vi "Label Targets Cones.vi"(5 "Details":bool, 7 "Annotate":bool=TRUE, 8 "Score Threshold":dbl, 9 "results":T1, 10 "Angle":dbl=53.2 format="%#_13g", 11 "Image in":T2) -> (3 "Image out":T2)   [LabVIEW 2025]
doc: "Draw scores near or on the particle and an ellipse around the target. Scores that are below the score threshold are drawn in red, above in green."
uses:
  <vilib>/vision/Image Controls.llb/IMAQ Image.ctl
  Target Fields.ctl
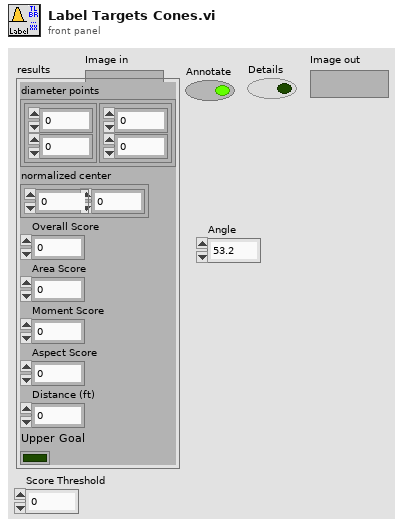
[diagram p1: front panel]
types:
  T1 = typedef "Target Fields.ctl" = cluster{"diameter points":cluster{"first point":cluster{"x":dbl, "y":dbl}, "projected point":cluster{"x":dbl, "y":dbl}}, "normalized center":cluster{"x":dbl, "y":dbl}, "Overall Score":dbl, "Area Score":dbl, "Moment Score":dbl, "Aspect Score":dbl, "Distance (ft)":dbl, "Upper Goal":bool}
  T2 = typedef "IMAQ Image.ctl" = refnum<image>
  T3 = cluster{"Desired Font (Application)":enum16{"User-specified Font", "Application Font", "System Font", "Dialog Font"}, "[User-specified Font]":cluster{"Font Name":string, "Size":i16, "Strikeout?":bool, "Italic?":bool, "Underline?":bool, "Outline?":bool, "Shadow?":bool, "Bold?":bool, "Rotation Angle":dbl}, "Horizontal Alignment":i16, "Vertical Alignment":i16}
  T4 = cluster{"first point":cluster{"x":dbl, "y":dbl}, "projected point":cluster{"x":dbl, "y":dbl}}
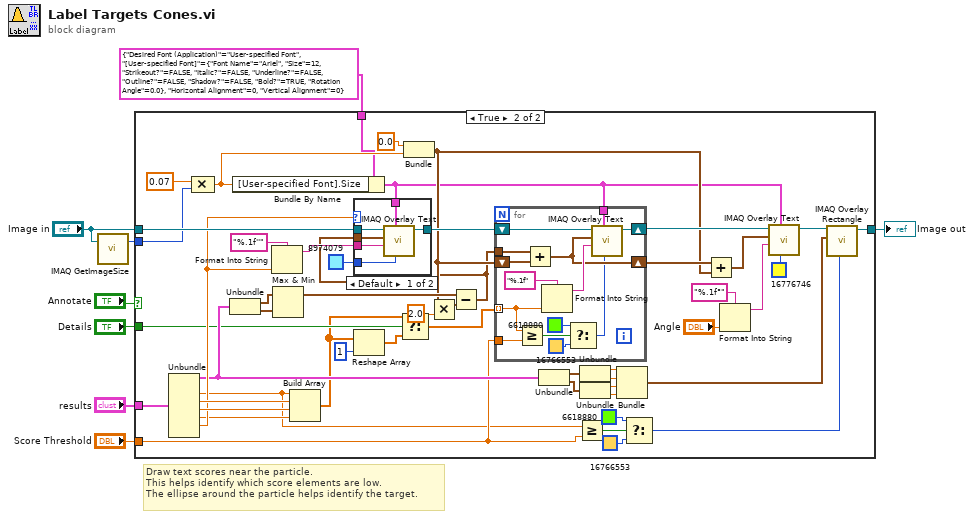
[diagram p0: block diagram]
diagram:
  # "Draw text scores near the particle.\nThis helps identify which score elements are low.\nThe ellipse around the particle helps identify the target."
  n1 = call "IMAQ GetImageSize"("Image"="Image in") -> ("Y Resolution"=w2:i32)  [unwired: 3 in, 2 out]
  n2 = case shown="True" "Annotate" {
    tunnel: [w9 w55] -> w8
    tunnel: "Image in" -> [w9 w60]
    tunnel: w2 -> [_ w27]
    tunnel: "results" -> [_ w56]
    tunnel: "Score Threshold" -> [_ w31]
    tunnel: "Details" -> [_ w38]
    tunnel: T3 {"Desired Font (Application)"=enum."User-specified Font", "[User-specified Font]"={"Font Name"="Ariel", "Size"=12, "Strikeout?"=FALSE, "Italic?"=FALSE, "Underline?"=FALSE, "Outline?"=FALSE, "Shadow?"=FALSE, "Bold?"=TRUE, "Rotation Angle"=0.0}, "Horizontal Alignment"=0, "Vertical Alignment"=0} ("Font, Size & Style") -> [_ w24]
    frame False {
    }
    frame True {
      n3 = Unbundle(w56) -> ("diameter points"=w46:T4, "Overall Score"=w30:dbl, "Area Score"=w54:dbl, "Moment Score"=w50:dbl, "Aspect Score"=w47:dbl, "Distance (ft)"=w48:dbl)  [unwired: 2 out]
      n4 = Compound Arithmetic op=MULTIPLY(0.07, w27) -> (w28:dbl)
      n5 = Unbundle(w46) -> ("first point"=w51:cluster{"x":dbl, "y":dbl}, "projected point"=w52:cluster{"x":dbl, "y":dbl})
      n6 = Bundle By Name(cluster=w24, "[User-specified Font].Size"=w28) -> (w13:T3)
      n7 = Format Into String(format string="%.1f''", w48) -> (resulting string=w59:string)  [unwired: 2 in, 1 out]
      n8 = Max & Min(x=w51, y=w52) -> (max(x,y)=w16:cluster{"x":dbl, "y":dbl})  [unwired: 1 out]
      n9 = Build Array(w30, w54, w50, w47) -> (w26:dbl[])
      n10 = Reshape Array(w26, 1) -> (w25:dbl[])
      n11 = Select(t=w26, s=w38, f=w25) -> (s? t:f=w37:dbl[])
      n12 = Bundle(0.0, w28) -> (w14:cluster{dbl, dbl})  [unwired: 1 in]
      n13 = Multiply(x=w14, y=2.0) -> (x*y=w11:cluster{dbl, dbl})
      n14 = Subtract(x=w16, y=w11) -> (x-y=w12:cluster{dbl, dbl})
      n15 = case shown="Default" w48 {
        tunnel: w60 -> [w80 w81]
        tunnel: w59 -> [w79 _]
        tunnel: w13 -> [w78 _]
        tunnel: [w77 w81] -> w53
        tunnel: w12 -> [w76 _]
        tunnel: u32 8974079 ("Color") -> [w75 _]
        frame Default {
          n16 = call "IMAQ Overlay Text"("Text Color (black)"=w75, "Font, Size & Style"=w78, "String"=w79, "Origin"=w76, "Image"=w80) -> ("Image Out"=w77:T2)  [unwired: 5 in, 1 out]
        }
        frame 0 {
        }
      }
      n17 = for {
        tunnel: w37 -> [w65] mode=indexing
        shift-right: [w71] -> w18
        shift-left: w53 -> [w72]
        tunnel: w13 -> [w70]
        shift-right: [w69] -> w17
        shift-left: w14 -> [w61]
        tunnel: w12 -> [w62]
        tunnel: w31 -> [w64]
        n18 = Greater Or Equal?(x=w65, y=w64) -> (x >= y?=w63:bool)
        n19 = Add(x=w62, y=w61) -> (x+y=w69:cluster{dbl, dbl})
        n20 = Format Into String(format string="%.1f", w65) -> (resulting string=w73:string)  [unwired: 2 in, 1 out]
        n21 = Select(t=u32 6618880 ("Color"), s=w63, f=u32 16766553 ("Color")) -> (s? t:f=w66:u32)
        n22 = call "IMAQ Overlay Text"("Text Color (black)"=w66, "Font, Size & Style"=w70, "String"=w73, "Origin"=w69, "Image"=w72) -> ("Image Out"=w71:T2)  [unwired: 5 in, 1 out]
      }
      n23 = Unbundle(w46) -> ("first point"=w45:cluster{"x":dbl, "y":dbl}, "projected point"=w44:cluster{"x":dbl, "y":dbl})
      n24 = Greater Or Equal?(x=w30, y=w31) -> (x >= y?=w32:bool)
      n25 = Unbundle(w45) -> ("x"=w43:dbl, "y"=w42:dbl)
      n26 = Unbundle(w44) -> ("x"=w41:dbl, "y"=w40:dbl)
      n27 = Bundle("x"=w43, "y"=w42, "x"=w41, "y"=w40) -> (w39:cluster{"x":dbl, "y":dbl, "x":dbl, "y":dbl})  [unwired: 1 in]
      n28 = Select(t=u32 6618880 ("Color"), s=w32, f=u32 16766553 ("Color")) -> (s? t:f=w33:u32)
      n29 = Add(x=w17, y=w14) -> (x+y=w19:cluster{dbl, dbl})
      n30 = Format Into String(format string="%.1f°", "Angle") -> (resulting string=w22:string)  [unwired: 2 in, 1 out]
      n31 = call "IMAQ Overlay Text"("Text Color (black)"=u32 16776746 ("Color"), "Font, Size & Style"=w13, "String"=w22, "Origin"=w19, "Image"=w18) -> ("Image Out"=w15:T2)  [unwired: 5 in, 1 out]
      n32 = call "IMAQ Overlay Rectangle"("Color"=w33, "Rectangle"=w39, "Image"=w15) -> ("Image Out"=w55:T2)  [unwired: 7 in, 1 out]
    }
  }
  "Image out" <- w8
